vi "IV to tsv 3 columns.vi"(8 "experiment name":string, 9 "Iteration":i32, 10 "Sweep parameters":T1, 11 "output cluster":cluster{dbl[], dbl[], dbl[]}) -> ()   [LabVIEW 2016]
uses:
  <vilib>/MakerHub/Toolbox/LMH-Toolbox.lvlib
panel:
  out "concatenated string":string
  out "appended path":path
  out "appended array":dbl[][](array[numeric])
  out "spreadsheet string":string
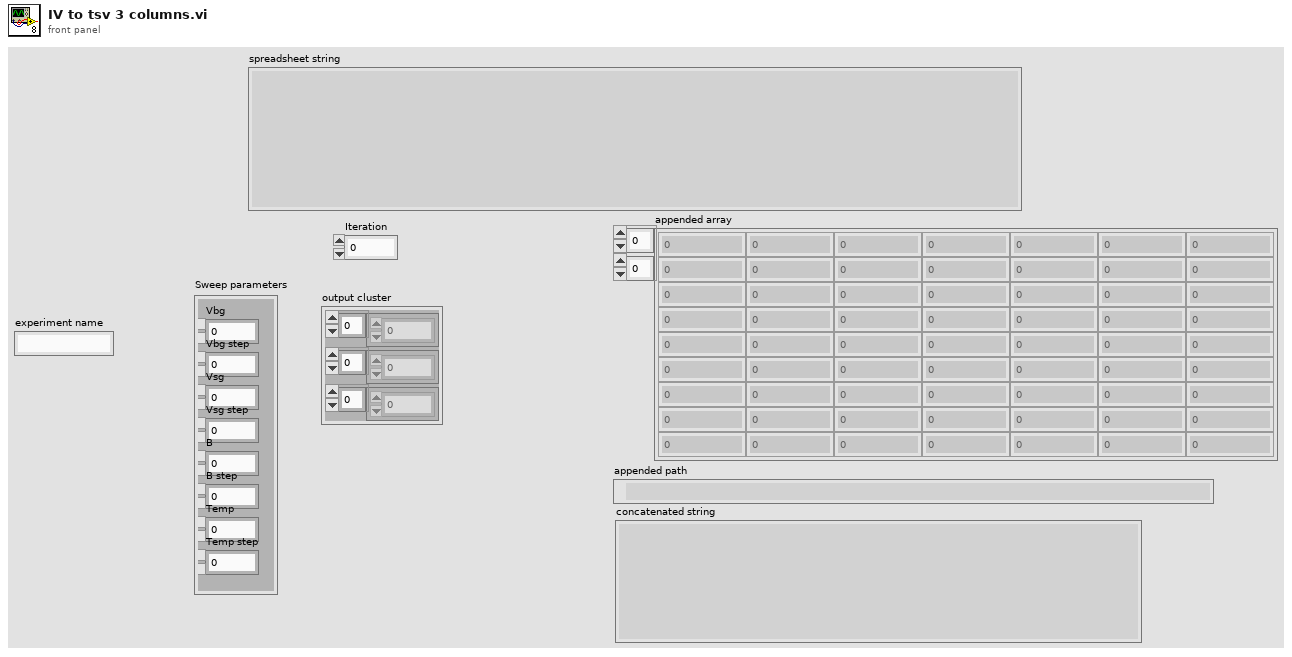
[diagram p1: front panel]
types:
  T1 = cluster{"Vbg":dbl, "Vbg step":dbl, "Vsg":dbl, "Vsg step":dbl, "B":dbl, "B step":dbl, "Temp":dbl, "Temp step":dbl}
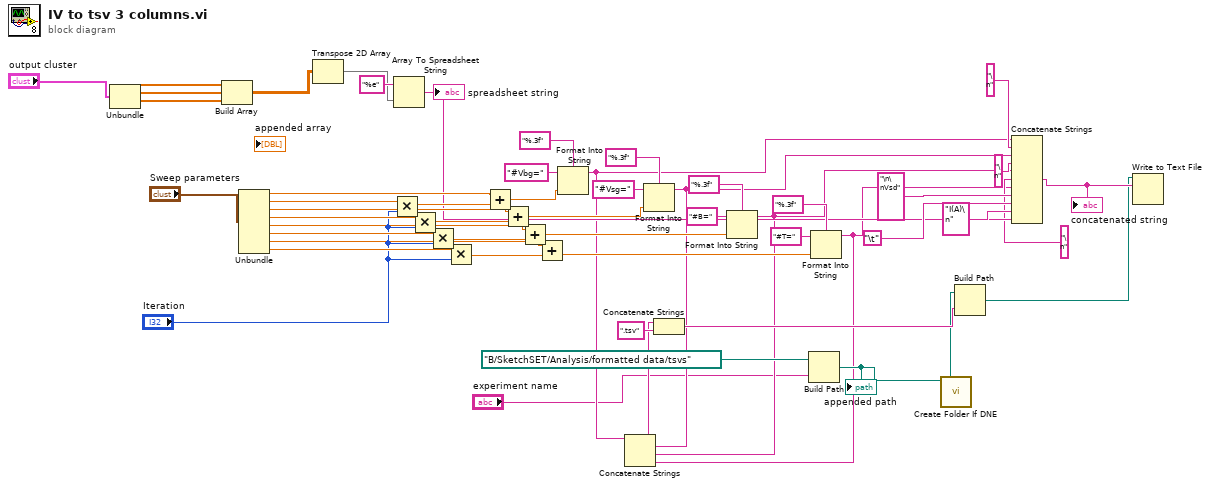
[diagram p0: block diagram]
diagram:
  n1 = Unbundle("output cluster") -> (w5:dbl[], w4:dbl[], w3:dbl[])
  n2 = Build Array(w5, w4, w3) -> (w2:dbl[][])
  n3 = Unbundle("Sweep parameters") -> ("Vbg"=w48:dbl, "Vbg step"=w52:dbl, "Vsg"=w46:dbl, "Vsg step"=w51:dbl, "B"=w44:dbl, "B step"=w50:dbl, "Temp"=w42:dbl, "Temp step"=w49:dbl)
  n4 = Transpose 2D Array(2D array=w2) -> (transposed array=w1:dbl[][])
  n5 = Multiply(x=w52, y="Iteration") -> (x*y=w47:dbl)
  n6 = Array To Spreadsheet String(array=w1, 3:"%e" ("format string")) -> (spreadsheet string=w26:string)  [unwired: 1 in]
  "spreadsheet string" <- w26
  n7 = Multiply(x=w51, y="Iteration") -> (x*y=w45:dbl)
  n8 = Multiply(x=w50, y="Iteration") -> (x*y=w43:dbl)
  n9 = Multiply(x=w49, y="Iteration") -> (x*y=w41:dbl)
  n10 = Add(x=w48, y=w47) -> (x+y=w39:dbl)
  n11 = Add(x=w46, y=w45) -> (x+y=w32:dbl)
  n12 = Add(x=w44, y=w43) -> (x+y=w31:dbl)
  n13 = Add(x=w42, y=w41) -> (x+y=w30:dbl)
  n14 = Format Into String(format string="%.3f", initial string="#Vbg=", w39) -> (resulting string=w14:string)  [unwired: 1 in, 1 out]
  n15 = Format Into String(format string="%.3f", initial string="#Vsg=", w32) -> (resulting string=w13:string)  [unwired: 1 in, 1 out]
  n16 = Format Into String(format string="%.3f", initial string="#B=", w31) -> (resulting string=w12:string)  [unwired: 1 in, 1 out]
  n17 = Build Path(base path=path "B:/SketchSET/Analysis/formatted data/tsvs", name or relative path="experiment name") -> (appended path=w19:path)
  "appended path" <- w19
  n18 = Format Into String(format string="%.3f", initial string="#T=", w30) -> (resulting string=w11:string)  [unwired: 1 in, 1 out]
  n19 = Concatenate Strings(w14, w13, w12, w11) -> (w10:string)
  n20 = Concatenate Strings(w10, ".tsv" ("string")) -> (w21:string)
  n21 = call <vilib>:"Create Folder If DNE.vi"("Folder Path"=w19) -> ("Dup Path"=w18:path)  [unwired: 9 in, 1 out]
  n22 = Build Path(base path=w18, name or relative path=w21) -> (appended path=w23:path)
  n23 = Concatenate Strings(w14, "\n" ("string"), w13, "\n" ("string"), w12, "\n" ("string"), w11, "\n\nVsd" ("string"), "\t", "I(A)\n" ("string"), w26) -> (w25:string)
  "concatenated string" <- w25
  n24 = Write to Text File(file (use dialog)=w23, text=w25) -> ()  [unwired: 2 in, 3 out]
